vi "LoadMenu.vi"(8 "error in (no error)":errorcluster, 11 "Menu in":refnum<class "Menu.lvclass">) -> (0 "error out":errorcluster, 3 "Menu out":refnum<class "Menu.lvclass">)   [LabVIEW 2021, in "Menu.lvlib" / "Menu.lvclass"]
uses:
  Menu.lvclass
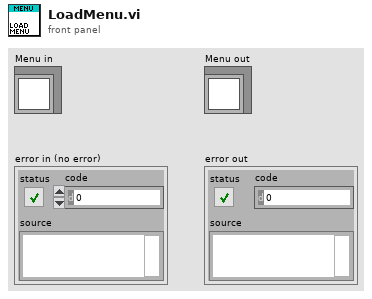
[diagram p1: front panel]
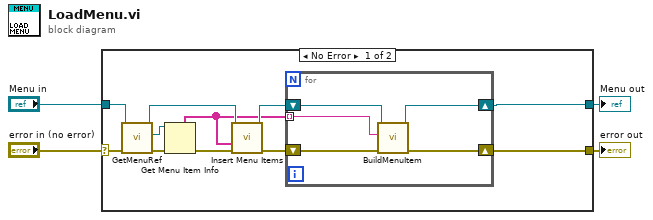
[diagram p0: block diagram]
diagram:
  n1 = case shown="No Error" "error in (no error)" {
    selector: "error in (no error)" -> [w12 w21]
    tunnel: [w14 w21] -> w4
    tunnel: "Menu in" -> [w10 w22]
    tunnel: [w13 w22] -> w2
    frame No Error {
      n2 = call "GetMenuRef.vi"("error in (no error)"=w12, "Menu in"=w10) -> ("error out"=w11:errorcluster, "RTMMenuReference"=w15:refnum<k9>, "Menu out"=w7:refnum<class "Menu.lvclass">)  [unwired: 7 in]
      n3 = Get Menu Item Info(8:w11, 11:w15) -> (0:w9:errorcluster, 5:w5:string[])  [unwired: 1 in, 5 out]
      n4 = call "Insert Menu Items.vi"("error in (no error)"=w9, "item tags"=w5, "Menu in"=w7) -> ("error out"=w8:errorcluster, "Menu out"=w6:refnum<class "Menu.lvclass">)  [unwired: 6 in, 1 out]
      n5 = for {
        tunnel: w5 -> [w18] mode=indexing
        shift-right: [w20] -> w14
        shift-left: w8 -> [w17]
        shift-right: [w19] -> w13
        shift-left: w6 -> [w16]
        n6 = call "BuildMenuItem.vi"("error"=w17, "ItemTag"=w18, "Menu"=w16) -> ("error out"=w20:errorcluster, "Menu out"=w19:refnum<class "Menu.lvclass">)  [unwired: 7 in]
      }
    }
    frame Error {
    }
  }
  "Menu out" <- w2
  "error out" <- w4
